vi "AO.vi"() -> ()   [LabVIEW 2021]
uses:
  <vilib>/userdefined/High Color/nirio_resource_hc.ctl
  <vilib>/FPGAPlugInAG/PCIe-7857/niLvFpga_Open_PCIe-7857.vi
  <vilib>/Utility/error.llb/Error Cluster From Error Code.vi
  <vilib>/rvi/errors/niLvFpgaAdjustHostInterfaceError.vi
  <vilib>/FPGAPlugInAG/PCIe-7857/niLvFpga_Close_PCIe-7857.vi
  <vilib>/rvi/interface/nirviOpenFPGA/nirviOpenFPGA.xnode
  FPGA Bitfiles/lvfpga2_FPGATarget_FPGA_J9MBVCOB9rw.lvbitx
  FPGA.vi
  <vilib>/rvi/interface/nirviReadWriteControl/nirviReadWriteControl.xnode
  <vilib>/rvi/interface/nirviCloseFPGA/nirviCloseFPGA.xnode
  NiFpgaLv.dll
panel:
  in  "RIO Resource Name":T1="RIO0" caption="RIO Device"
  in  "stop":bool
  in  "AO Channels":dbl[](array[slide]) scale=-10.0..9.995 scale format="%.1f"
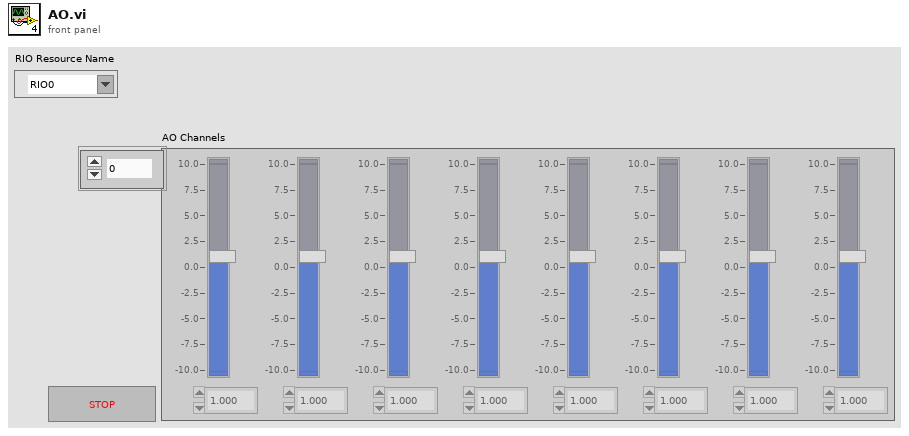
[diagram p1: front panel]
types:
  T1 = typedef "nirio_resource_hc.ctl" = tag
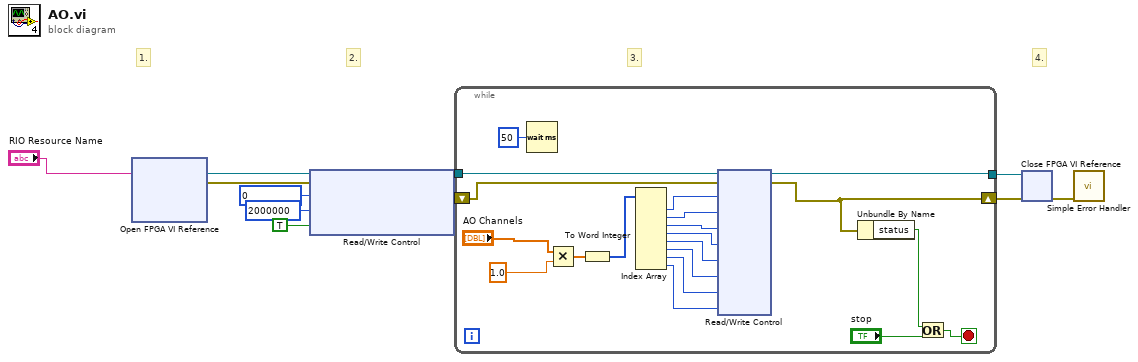
[diagram p0: block diagram]
diagram:
  # "4."
  # "3."
  # "2."
  # "1."
  n1 = xnode "Open FPGA VI Reference"("resource name"="RIO Resource Name") -> ("FPGA VI Reference Out"=w8:refnum<k20>, "error out"=w7:errorcluster)  [unwired: 1 in]
  n2 = xnode "Read/Write Control"("FPGA VI Reference In"=w8, "error in"=w7, "AO Buffer Enable"=u8 0, "AO Loop Timer(Ticks)"=u32 2000000, "AO Enable"=TRUE) -> ("FPGA VI Reference Out"=w6:refnum<k20>, "error out"=w5:errorcluster)
  n3 = while {
    tunnel: w6 -> [w31]
    shift-right: [w13] -> w10
    shift-left: w5 -> [w30]
    tunnel: [w14] -> w11
    stop <- w15 stop-if-true
    n4 = Wait (ms)(milliseconds to wait=u32 50) -> ()  [unwired: 1 out]
    n5 = Multiply(x="AO Channels", y=1.0) -> (x*y=w20:dbl[])
    n6 = To Word Integer(number=w20) -> (16bit integer=w19:i16[])
    n7 = Index Array(array=w19) -> (element #1=w28:i16, element #2=w27:i16, element #3=w26:i16, element #4=w25:i16, element #5=w24:i16, element #6=w23:i16, element #7=w22:i16, element #8=w21:i16)  [unwired: 8 in]
    n8 = xnode "Read/Write Control"("FPGA VI Reference In"=w31, "error in"=w30, "AO 0"=w28, "AO 1"=w27, "AO 2"=w26, "AO 3"=w25, "AO 4"=w24, "AO 5"=w23, "AO 6"=w22, "AO 7"=w21) -> ("FPGA VI Reference Out"=w14:refnum<k20>, "error out"=w13:errorcluster)
    n9 = Unbundle By Name(w13) -> ("status"=w16:bool)
    n10 = Or(x=w16, y="stop") -> (x .or. y?=w15:bool)
  }
  n11 = xnode "Close FPGA VI Reference"("FPGA VI Reference In"=w11, "error in"=w10) -> ("error out"=w9:errorcluster)
  n12 = call <vilib>:"Simple Error Handler.vi"("error in (no error)"=w9) -> ()  [unwired: 4 in, 5 out]
